vi "GetStringPropertyValue.vi"(0 ".NET Refnum":refnum<k24>) -> (1 ".NET Refnum Out":refnum<k24>, 2 "String Value Property":string, 3 "error out":errorcluster)   [LabVIEW 2012]
uses:
  D:/tsdev/Tests/LVBuildValidation/12.0/Automated/FlexLVAdapter30/Refnums/DotNetRefnum/LabviewDNTest.dll
  LabviewDNTest.dll
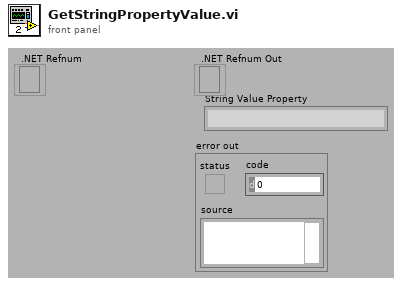
[diagram p1: front panel]
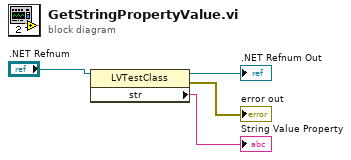
[diagram p0: block diagram]
diagram:
  n1 = property class="LVTestClass"(reference=".NET Refnum") -> (reference out=→".NET Refnum Out":refnum<k24>, error out=→"error out":errorcluster, "str"=→"String Value Property":string)  [unwired: 1 in]
